vi "obstacle avoidance.vi"   [LabVIEW 2009]
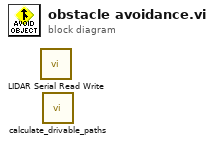
[diagram p0: block diagram]
diagram:
  n1 = call "LIDAR Serial Read Write.vi"() -> ()  [unwired: 1 in]
  n2 = call "calculate_drivable_paths.vi"() -> ()  [unwired: 1 in]
